vi "get_modifier_base_value.vi"(8 "error in (no error)":errorcluster, 10 "modifier index":i32, 11 "GenericTrajectory.lvclass in":refnum<class "TrajectoryDL091126GenericVoxel.lvclass">) -> (0 "error out":errorcluster, 2 "intensity modifier base value":dbl, 3 "GenericTrajectory.lvclass out":refnum<class "TrajectoryDL091126GenericVoxel.lvclass">)   [LabVIEW 2010, in "TrajectoryDL091126GenericVoxel.lvclass"]
uses:
  TrajectoryDL091126GenericVoxel.lvclass
  TrajectoryDL091126GenericVoxel.lvclass/TrajectoryDL091126GenericVoxel.ctl
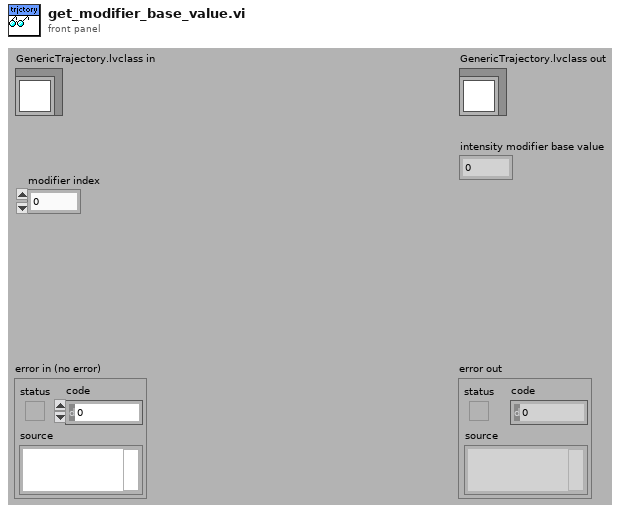
[diagram p1: front panel]
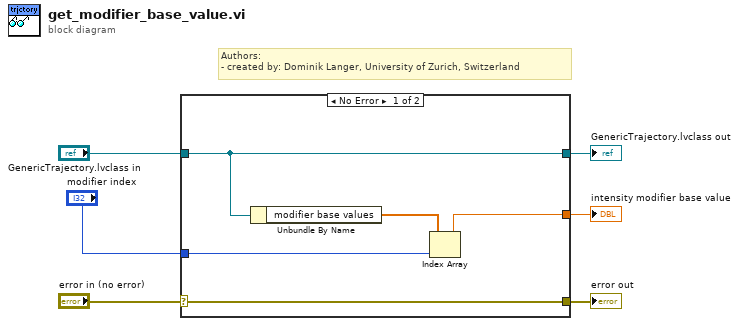
[diagram p0: block diagram]
diagram:
  # "Authors: \n- created by: Dominik Langer, University of Zurich, Switzerland"
  n1 = case shown="No Error" "error in (no error)" {
    selector: "error in (no error)" -> [w11 w12]
    tunnel: [w11 w12] -> w5
    tunnel: [w10 w13] -> w3
    tunnel: "GenericTrajectory.lvclass in" -> [w10 w13]
    tunnel: [w8 _] -> w2
    tunnel: "modifier index" -> [w7 _]
    frame No Error {
      n2 = Unbundle By Name(w10) -> ("modifier base values"=w9:dbl[])
      n3 = Index Array(array=w9, index=w7) -> (element=w8:dbl)
    }
    frame Error {
    }
  }
  "error out" <- w5
  "GenericTrajectory.lvclass out" <- w3
  "intensity modifier base value" <- w2
